vi "AIT 664 - Write outgoing message data.vi"(0 "Driver Data":T4 {"Num Bits" min=1 max=32}, 5 "Values":dbl[](array[numeric]), 7 "Channel Index":i32, 9 "Msg Data In":u8[](array[numeric]), 11 "error in (no error)":errorcluster, 12 "Iteration":i32, 13 "Tx Com Udp Port":T1 {"Handle" format="%08x"}) -> (10 "Msg Data Out":u8[](array[numeric]), 15 "error out":errorcluster)   [LabVIEW 2013, in "AIT 664 Custom Device.lvlib"]
doc: "Convert double array to U8 array and send out AIT 664 card"
uses:
  AIT 664 Custom Device.lvlib
  RT Controls/AIT 664 - Driver Data.ctl
  Controls and Global/Start Bit.ctl
  Controls and Global/Number of Bits.ctl
  <userlib>/ARINC 664/AIT 664 Controls/General/Message Port.ctl
  <userlib>/ARINC 664/AIT 664 Controls/General/Direction.ctl
  <userlib>/ARINC 664/AIT 664 Controls/General/Message Port Type.ctl
  System Explorer/Controls/664 -Param.ctl
  <instrlib>/AIT 664/Private/AIT 664 Data/Tx/Write/AIT 664 Tx Write (ComUdp).vi
  <vilib>/NI Veristand/Custom Device Tools/Custom Device Utility Library/Custom Device Utility Library.lvlib
  <instrlib>/AIT 664/AIT 664.lvlib
  <userlib>/ARINC 664/AIT 664 API.lvlib
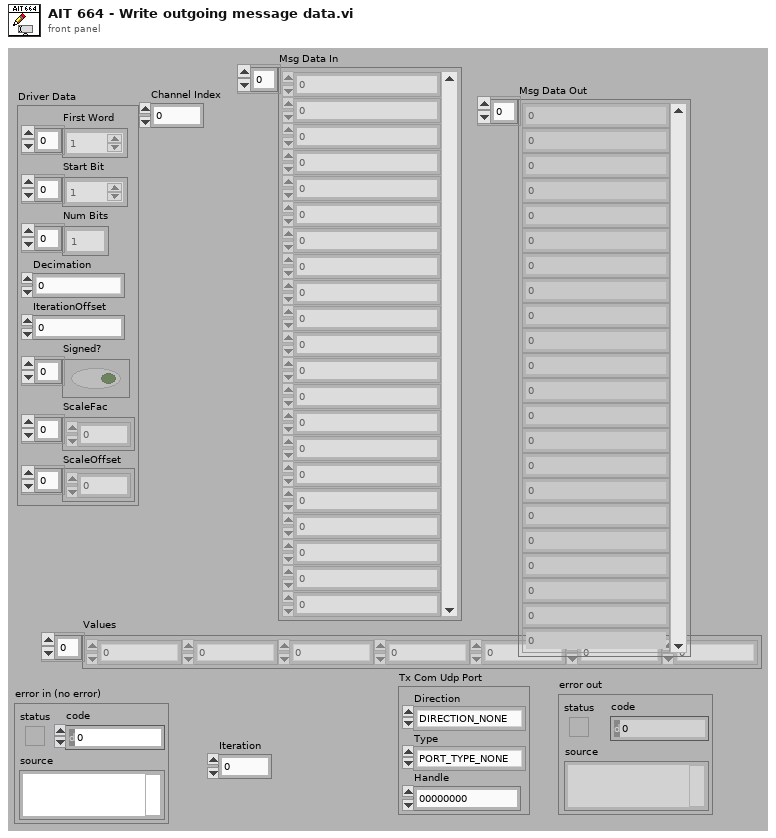
[diagram p1: front panel]
types:
  T1 = typedef "AIT 664 API.lvlib/Message Port.ctl" = cluster{"Direction":T2, "Type":T3, "Handle":u64}
  T2 = typedef "AIT 664 API.lvlib/Direction.ctl" = enum16{"DIRECTION_NONE", "DIRECTION_TX", "DIRECTION_RX"}
  T3 = typedef "AIT 664 API.lvlib/Message Port Type.ctl" = enum16{"PORT_TYPE_NONE", "COM_UDP", "SAP_UDP", "SAP_IP", "SAP_MAC", "COTS_MAC", "COTS_MAC_RAW"}
  T4 = typedef "AIT 664 Custom Device.lvlib/AIT 664 - Driver Data.ctl" = cluster{"First Word":T5[], "Start Bit":T5[], "Num Bits":T6[], "Decimation":i32, "IterationOffset":i32, "Signed?":bool[], "ScaleFac":dbl[], "ScaleOffset":dbl[]}
  T5 = typedef "AIT 664 Custom Device.lvlib/Start Bit.ctl" = i32
  T6 = typedef "AIT 664 Custom Device.lvlib/Number of Bits.ctl" = i32
  T7 = typedef "AIT 664 Custom Device.lvlib/664 -Param.ctl" = cluster{"name":string, "firstByte":i32, "startBit":i32, "numberBits":i32, "scaleFactor":dbl, "scaleOffset":dbl, "signed":bool}
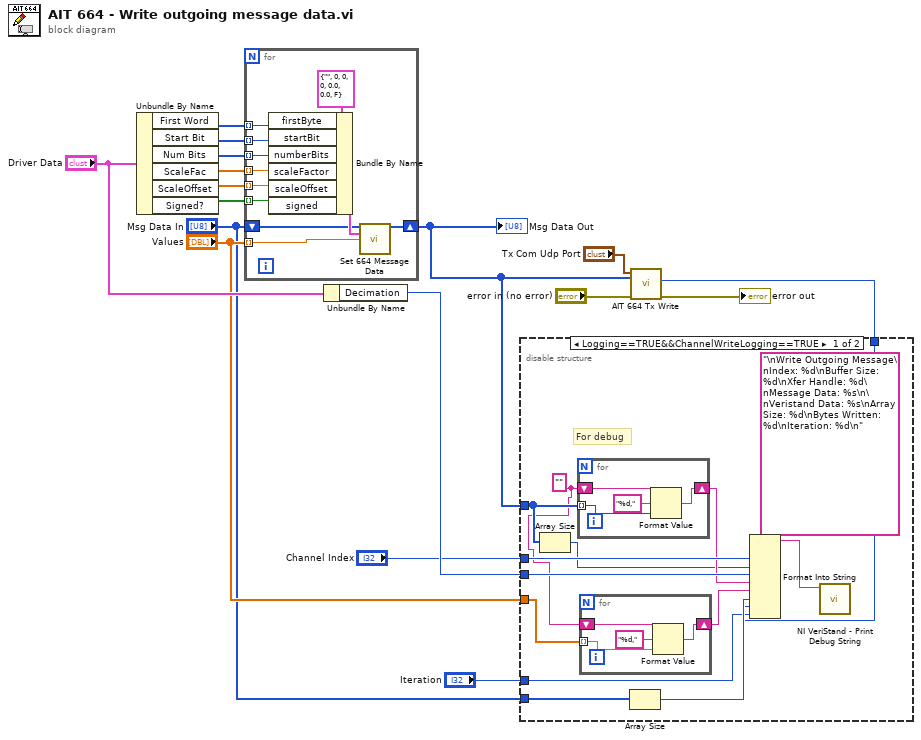
[diagram p0: block diagram]
diagram:
  n1 = Unbundle By Name("Driver Data") -> ("First Word"=w5:T5[], "Start Bit"=w17:T5[], "Num Bits"=w4:T6[], "ScaleFac"=w16:dbl[], "ScaleOffset"=w15:dbl[], "Signed?"=w14:bool[])
  n2 = for {
    tunnel: w5 -> [w27] mode=indexing
    tunnel: w17 -> [w26] mode=indexing
    tunnel: w4 -> [w25] mode=indexing
    tunnel: w16 -> [w24] mode=indexing
    tunnel: w15 -> [w23] mode=indexing
    tunnel: w14 -> [w22] mode=indexing
    tunnel: "Values" -> [w19] mode=indexing
    shift-right: [w18] -> w8
    shift-left: "Msg Data In" -> [w20]
    n3 = Bundle By Name(cluster=T7 {"name"="", "firstByte"=0, "startBit"=0, "numberBits"=0, "scaleFactor"=0.0, "scaleOffset"=0.0, "signed"=FALSE} ("1553 Parameter"), "firstByte"=w27, "startBit"=w26, "numberBits"=w25, "scaleFactor"=w24, "scaleOffset"=w23, "signed"=w22) -> (w21:T7)
    n4 = call "Set 664 Message Data.vi"("MSG DATA In"=w20, "664 Parameter"=w21, "Value"=w19) -> ("MSG DATA Out"=w18:u8[])  [unwired: 11 in, 1 out]
  }
  "Msg Data Out" <- w8
  n5 = Unbundle By Name("Driver Data") -> ("Decimation"=w12:i32)
  n6 = call-poly <instrlib>:"AIT 664 Tx Write.vi"("error in"="error in (no error)", "Tx Com Udp Data in"=w8, "Tx Com Udp Port in"="Tx Com Udp Port") -> ("error out"=→"error out":errorcluster, "Bytes Written out"=w2:u16)  [unwired: 4 in, 1 out]
  n7 = disable-structure shown="Logging==TRUE&&ChannelWriteLogging==TRUE" {
    disable-tunnel: w8 -> [w37 _]
    disable-tunnel: "Channel Index" -> [w42 _]
    disable-tunnel: w12 -> [w41 _]
    disable-tunnel: "Values" -> [w35 _]
    disable-tunnel: "Msg Data In" -> [w32 _]
    disable-tunnel: w2 -> [w30 _]
    disable-tunnel: "Iteration" -> [w29 _]
    frame condition #0 (active) {
      w34 = "" ("format string")
      # "For debug"
      n8 = Array Size(array=w37) -> (size(s)=w36:i32)
      n9 = for {
        tunnel: w37 -> [w47] mode=indexing
        shift-right: [w48] -> w39
        shift-left: w34 -> [w49]
        n10 = Format Value(string ("")=w49, format string="%d,", value (0)=w47) -> (output string=w48:string)
      }
      n11 = for {
        tunnel: w35 -> [w43] mode=indexing
        shift-right: [w44] -> w33
        shift-left: w34 -> [w45]
        n12 = Format Value(string ("")=w45, format string="%d,", value (0)=w43) -> (output string=w44:string)
      }
      n13 = Array Size(array=w32) -> (size(s)=w31:i32)
      n14 = Format Into String(format string="\nWrite Outgoing Message\nIndex: %d\nBuffer Size: %d\nXfer Handle: %d\nMessage Data: %s\n\nVeristand Data: %s\nArray Size: %d\nBytes Written: %d\nIteration: %d\n", w42, w36, w41, w39, w33, w31, w30, w29) -> (resulting string=w38:string)  [unwired: 2 in, 1 out]
      n15 = call <vilib>:"NI VeriStand - Print Debug String.vi"("Message"=w38) -> ()  [unwired: 10 in, 1 out]
    }
    frame condition #1 {
    }
  }
